vi "InterfaceControladores2.vi"() -> ()   [LabVIEW 2016]
uses:
  <vilib>/Instr/_visa.llb/VISA Configure Serial Port (Instr).vi
panel:
  out "u":dbl
  in  "Tab Control":T1(tab)
  out "Error Signal":dbl(graph)
  out "Control Signal":dbl(graph)
  out "Referece Signal":dbl(graph)
  out "Output Signal":dbl(graph)
  in  "Send":bool
  in  "Fuzzy Input Launcher 2":bool
  in  "Fuzzy Input Launcher":bool
  in  "Send 2":bool
  in  "PORT":refnum<visa-resource-name>
  in  "Controller":u16(ring) items=["On/Off", "On/Off Hysteresis", "Proportional", "Proportional Integral", "Fuzzy", "Open Loop"]
  in  "Reference (V)":dbl(slide) min=0.0 max=20.0 scale=0.0..20.0
  in  "Window Hysteresis %":dbl min=0.0 max=99.0
  in  "Kp":dbl(knob) min=-1.0 max=10.0 scale=-1.0..10.0 scale format="%.1g"
  in  "Ki":dbl(knob) min=0.0 max=10.0 scale=0.0..10.0 scale format="%.1g"
  in  "Stop Button":bool
  out "data sent":string
  out "y":dbl
  # "P/PI Controller"
  # "On/Off with Hysteresis Controller"
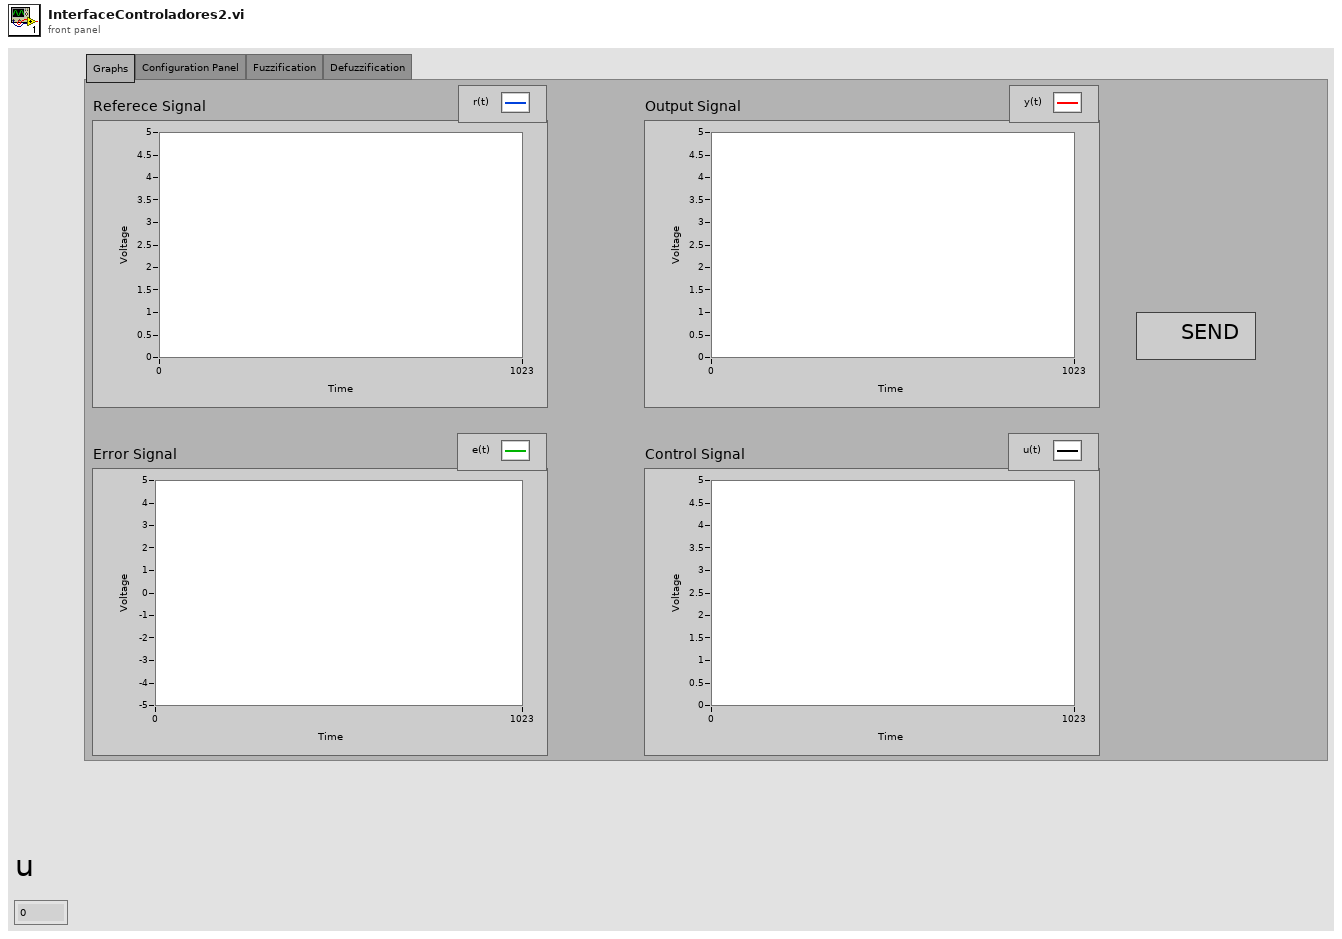
[diagram p1: front panel]
types:
  T1 = enum32{"Graphs", "Configuration Panel", "Fuzzification", "Defuzzification"}
  T2 = enum32{"Invalid", "Standard", "Closed", "Hidden", "Minimized", "Maximized"}
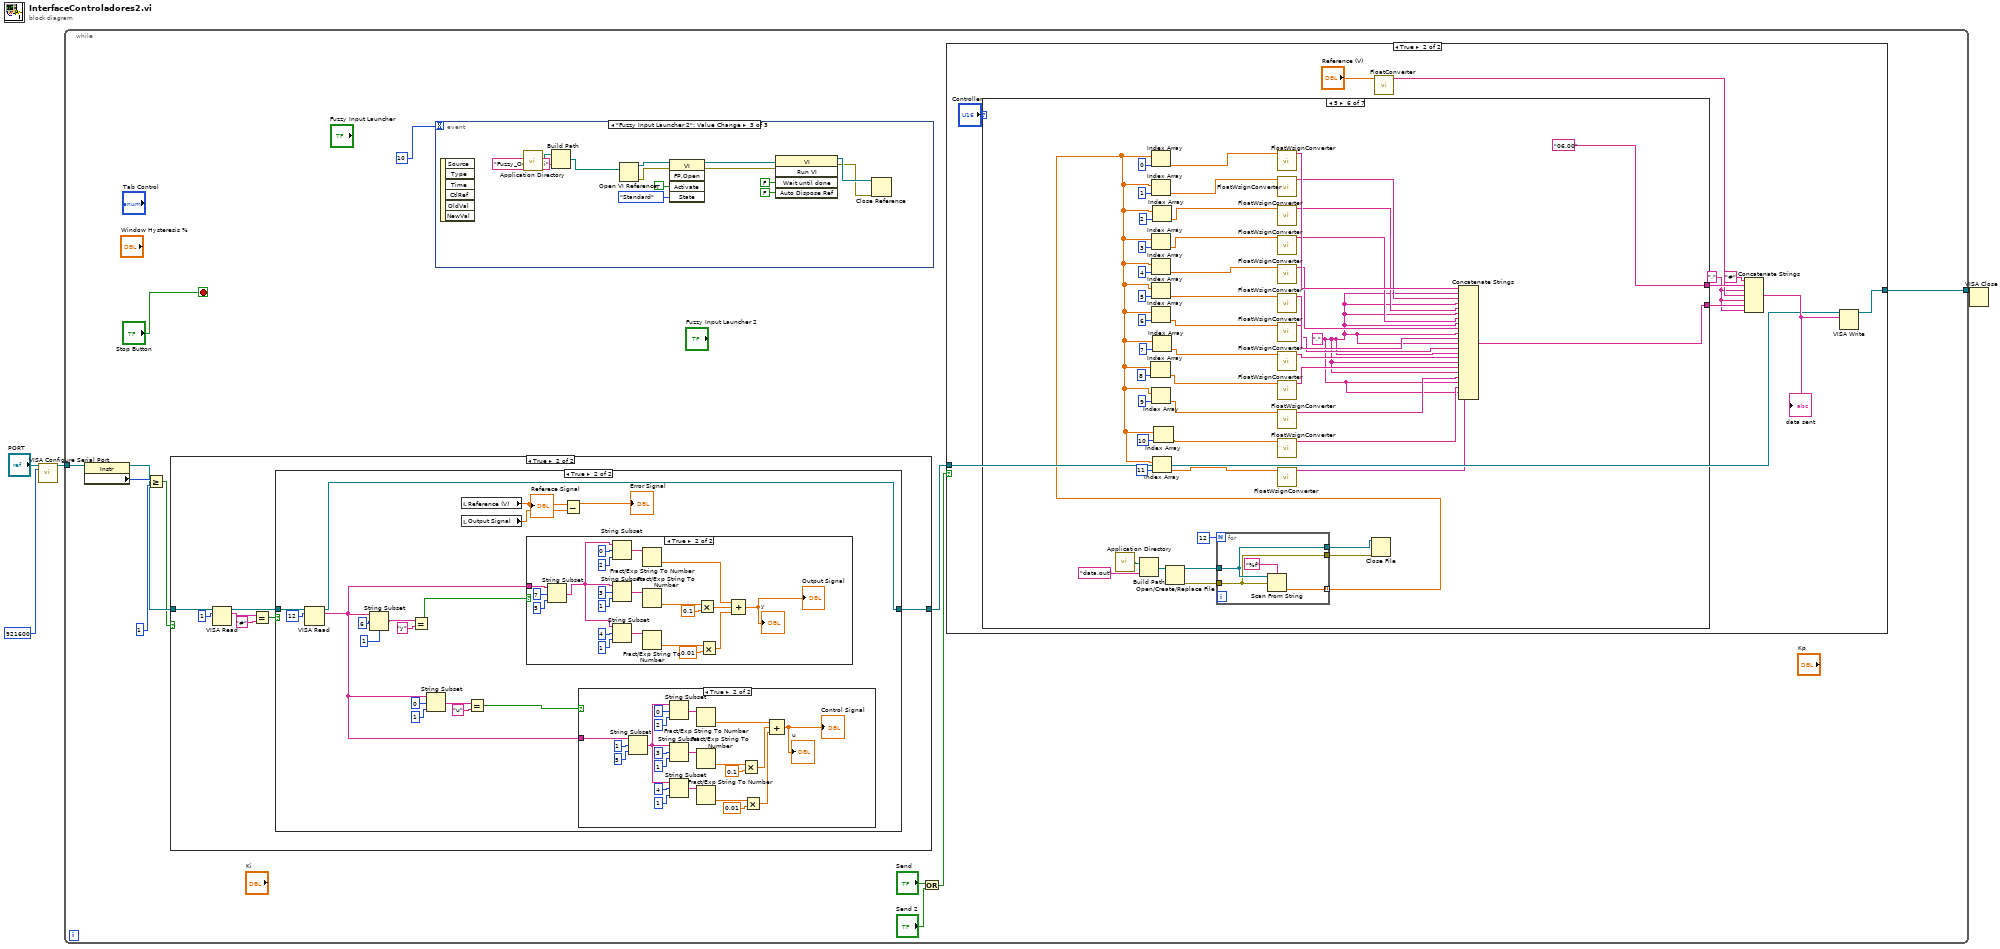
[diagram p0: block diagram]
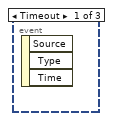
[diagram p2: hidden frame]
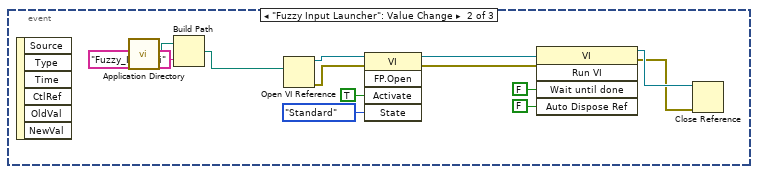
[diagram p3: hidden frame]
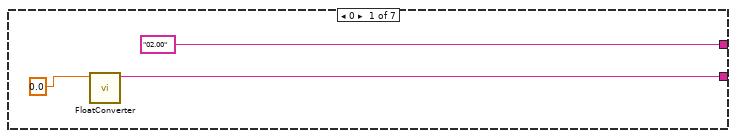
[diagram p9: hidden frame]
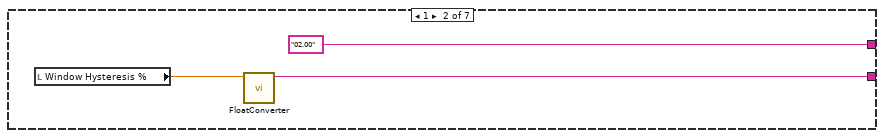
[diagram p10: hidden frame]
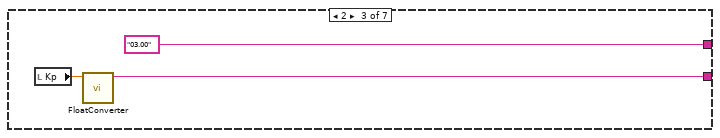
[diagram p11: hidden frame]
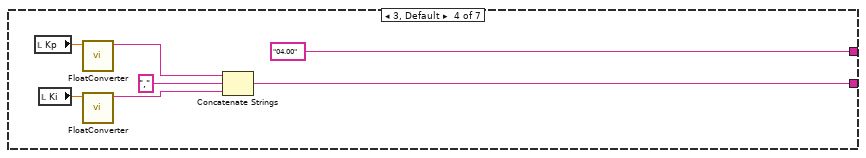
[diagram p12: hidden frame]
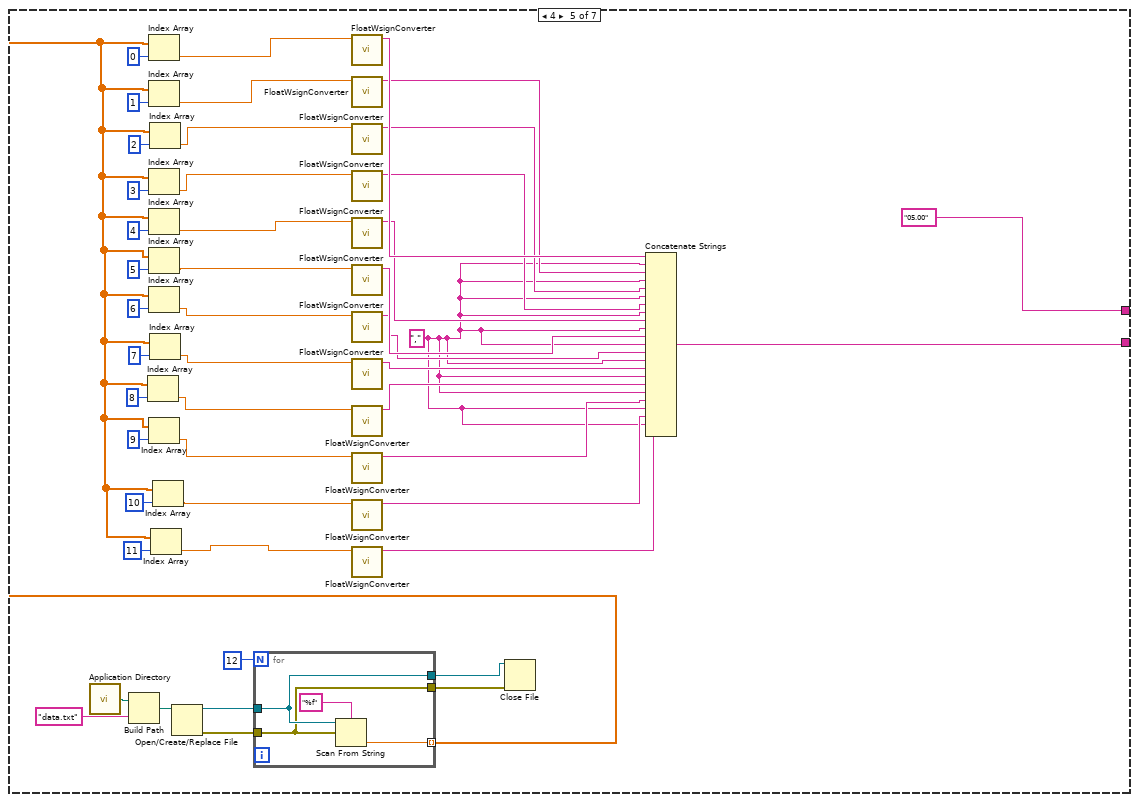
[diagram p13: hidden frame]
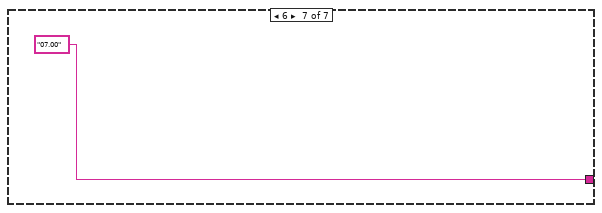
[diagram p14: hidden frame]
diagram:
  n1 = call-poly "VISA Configure Serial Port"("VISA resource name"="PORT", "baud rate (9600)"=u32 921600) -> ("VISA resource name out"=w4:refnum<visa-resource-name>)  [unwired: 12 in, 1 out]
  n2 = while {
    tunnel: w4 -> [w16]
    tunnel: [w13] -> w2
    stop <- "Stop Button" stop-if-true
    n3 = property class="Instr"(reference=w16) -> (reference out=w12:refnum<visa-resource-name>, "Serial Settings:Number of Bytes at Serial Port"=w15:u32)  [unwired: 1 in, 1 out]
    n4 = Greater Or Equal?(x=w15, y=u32 1) -> (x >= y?=w11:bool)
    n5 = case shown="True" w11 {
      tunnel: w12 -> [w43 w50]
      tunnel: [w43 w44] -> w10
      frame False {
      }
      frame True {
        n6 = VISA Read(VISA resource name=w50, byte count=u32 1 ("y")) -> (VISA resource name out=w45:refnum<visa-resource-name>, read buffer=w48:string)  [unwired: 1 in, 2 out]
        n7 = Equal?(x=w48, y="#") -> (x = y?=w46:bool)
        n8 = case shown="True" w46 {
          tunnel: [w51 w67] -> w44
          tunnel: w45 -> [w51 w66]
          frame False {
          }
          frame True {
            n9 = VISA Read(VISA resource name=w66, byte count=u32 12 ("y")) -> (VISA resource name out=w67:refnum<visa-resource-name>, read buffer=w52:string)  [unwired: 1 in, 2 out]
            n10 = String Subset(string=w52, offset (0)=6 ("length (rest)"), length (rest)=1 ("length (rest)")) -> (substring=w55:string)
            n11 = Equal?(x=w55, y="y") -> (x = y?=w54:bool)
            n12 = String Subset(string=w52, offset (0)=0 ("length (rest)"), length (rest)=1 ("length (rest)")) -> (substring=w57:string)
            n13 = local read "Reference (V)"() -> (w64:dbl)
            "Referece Signal" <- w64
            n14 = local read "Output Signal"() -> (w65:dbl)
            n15 = Equal?(x=w57, y="u") -> (x = y?=w53:bool)
            n16 = case shown="True" w54 {
              tunnel: w52 -> [_ w70]
              frame False {
              }
              frame True {
                n17 = String Subset(string=w70, offset (0)=7, length (rest)=5 ("length (rest)")) -> (substring=w69:string)
                n18 = String Subset(string=w69, offset (0)=0, length (rest)=2 ("length (rest)")) -> (substring=w88:string)
                n19 = String Subset(string=w69, offset (0)=3, length (rest)=1 ("length (rest)")) -> (substring=w87:string)
                n20 = String Subset(string=w69, offset (0)=4, length (rest)=1 ("offset (0)")) -> (substring=w79:string)
                n21 = Fract/Exp String To Number(string=w88) -> (number=w76:dbl)  [unwired: 3 in, 1 out]
                n22 = Fract/Exp String To Number(string=w87) -> (number=w84:dbl)  [unwired: 3 in, 1 out]
                n23 = Fract/Exp String To Number(string=w79) -> (number=w80:dbl)  [unwired: 3 in, 1 out]
                n24 = Multiply(x=w84, y=0.1) -> (x*y=w75:dbl)
                n25 = Multiply(x=w80, y=0.01) -> (x*y=w74:dbl)
                n26 = Compound Arithmetic op=ADD(w76, w75, w74) -> (→"Output Signal" →"y":dbl)
              }
            }
            n27 = Subtract(x=w64, y=w65) -> (x-y=→"Error Signal":dbl)
            n28 = case shown="True" w53 {
              tunnel: w52 -> [_ w93]
              frame False {
              }
              frame True {
                n29 = String Subset(string=w93, offset (0)=1, length (rest)=5 ("length (rest)")) -> (substring=w94:string)
                n30 = String Subset(string=w94, offset (0)=0, length (rest)=2 ("offset (0)")) -> (substring=w109:string)
                n31 = String Subset(string=w94, offset (0)=3, length (rest)=1 ("offset (0)")) -> (substring=w107:string)
                n32 = String Subset(string=w94, offset (0)=4, length (rest)=1 ("offset (0)")) -> (substring=w100:string)
                n33 = Fract/Exp String To Number(string=w109) -> (number=w98:dbl)  [unwired: 3 in, 1 out]
                n34 = Fract/Exp String To Number(string=w107) -> (number=w106:dbl)  [unwired: 3 in, 1 out]
                n35 = Fract/Exp String To Number(string=w100) -> (number=w101:dbl)  [unwired: 3 in, 1 out]
                n36 = Multiply(x=w106, y=0.1) -> (x*y=w97:dbl)
                n37 = Multiply(x=w101, y=0.01) -> (x*y=w96:dbl)
                n38 = Compound Arithmetic op=ADD(w98, w97, w96) -> (→"Control Signal" →"u":dbl)
              }
            }
          }
        }
      }
    }
    n39 = event shown="[2] \"Fuzzy Input Launcher 2\": Value Change" {
      selector: _ -> [_ _ _]
      dyn-events: _ -> [_ _ _]
      timeout: 10 -> [_ _ _]
      event Timeout {
        n40 = event-data() -> ()  [unwired: 1 in, 3 out]
      }
      event "Fuzzy Input Launcher": Value Change {
        n41 = event-data() -> ()  [unwired: 1 in, 6 out]
        n42 = call <vilib>:"Application Directory.vi"() -> ("Application Directory"=w29:path)
        n43 = Build Path(base path=w29, name or relative path="Fuzzy_Input.vi") -> (appended path=w27:path)
        n44 = Open VI Reference(vi path=w27) -> (vi reference=w24:refnum<vi>, error out=w23:errorcluster)  [unwired: 5 in]
        n45 = invoke class="VI" method="FP.Open"(reference=w24, error in=w23, "Activate"=TRUE ("Activate?"), "State"=T2."Standard") -> (reference out=w26:refnum<vi>, error out=w25:errorcluster)  [unwired: 1 in, 3 out]
        n46 = invoke class="VI" method="Run VI"(reference=w26, error in=w25, "Wait until done"=FALSE ("Wait Until Done"), "Auto Dispose Ref"=FALSE ("Auto Dispose Reference")) -> (reference out=w18:refnum<vi>, error out=w17:errorcluster)  [unwired: 1 in, 3 out]
        n47 = Close Reference(reference=w18, error in (no error)=w17) -> ()  [unwired: 1 out]
      }
      event "Fuzzy Input Launcher 2": Value Change {
        n48 = event-data() -> ()  [unwired: 1 in, 6 out]
        n49 = call <vilib>:"Application Directory.vi"() -> ("Application Directory"=w42:path)
        n50 = Build Path(base path=w42, name or relative path="Fuzzy_Output.vi") -> (appended path=w40:path)
        n51 = Open VI Reference(vi path=w40) -> (vi reference=w37:refnum<vi>, error out=w36:errorcluster)  [unwired: 5 in]
        n52 = invoke class="VI" method="FP.Open"(reference=w37, error in=w36, "Activate"=TRUE ("Activate?"), "State"=T2."Standard") -> (reference out=w39:refnum<vi>, error out=w38:errorcluster)  [unwired: 1 in, 3 out]
        n53 = invoke class="VI" method="Run VI"(reference=w39, error in=w38, "Wait until done"=FALSE ("Wait Until Done"), "Auto Dispose Ref"=FALSE ("Auto Dispose Reference")) -> (reference out=w31:refnum<vi>, error out=w30:errorcluster)  [unwired: 1 in, 3 out]
        n54 = Close Reference(reference=w31, error in (no error)=w30) -> ()  [unwired: 1 out]
      }
    }
    n55 = Or(x="Send", y="Send 2") -> (x .or. y?=w7:bool)
    n56 = case shown="True" w7 {
      tunnel: [w111 w119] -> w13
      tunnel: w10 -> [w111 w117]
      frame False {
      }
      frame True {
        w112 = ","
        n57 = case shown="5" "Controller" {
          tunnel: [w123 w125 w128 w136 w138 w190 _] -> w113
          tunnel: ["02.00" "02.00" "03.00" "04.00" "05.00" "06.00" "07.00"] -> w115
          frame 0 {
            n58 = call "FloatConverter.vi"("Reference (V)"=0.0) -> ("String"=w123:string)  [unwired: 10 in]
          }
          frame 1 {
            n59 = local read "Window Hysteresis %"() -> (w126:dbl)
            n60 = call "FloatConverter.vi"("Reference (V)"=w126) -> ("String"=w125:string)  [unwired: 10 in]
          }
          frame 2 {
            n61 = local read "Kp"() -> (w129:dbl)
            n62 = call "FloatConverter.vi"("Reference (V)"=w129) -> ("String"=w128:string)  [unwired: 10 in]
          }
          frame 3, Default {
            n63 = local read "Kp"() -> (w134:dbl)
            n64 = local read "Ki"() -> (w132:dbl)
            n65 = call "FloatConverter.vi"("Reference (V)"=w134) -> ("String"=w133:string)  [unwired: 10 in]
            n66 = call "FloatConverter.vi"("Reference (V)"=w132) -> ("String"=w131:string)  [unwired: 10 in]
            n67 = Concatenate Strings(w133, ",", w131) -> (w136:string)
          }
          frame 4 {
            w140 = ","
            n68 = call <vilib>:"Application Directory.vi"() -> ("Application Directory"=w183:path)
            n69 = Build Path(base path=w183, name or relative path="data.txt") -> (appended path=w177:path)
            n70 = Open/Create/Replace File(file path (use dialog)=w177) -> (refnum out=w181:refnum<file>, error out=w180:errorcluster)  [unwired: 5 in, 1 out]
            n71 = for {
              N: 12 -> [_]
              tunnel: w181 -> [w187]
              tunnel: w180 -> [w186]
              tunnel: [w188] -> w164 mode=indexing
              tunnel: [w187] -> w179
              tunnel: [w186] -> w178
              n72 = Scan From String("%f" ("format string"), w187, w186) -> (output 1=w188:dbl)  [unwired: 1 in, 2 out]
            }
            n73 = Index Array(array=w164, index=8) -> (element=w155:dbl)
            n74 = Index Array(array=w164, index=0) -> (element=w163:dbl)
            n75 = Index Array(array=w164, index=1) -> (element=w162:dbl)
            n76 = Index Array(array=w164, index=3) -> (element=w160:dbl)
            n77 = Index Array(array=w164, index=4) -> (element=w159:dbl)
            n78 = Index Array(array=w164, index=5) -> (element=w158:dbl)
            n79 = Index Array(array=w164, index=6) -> (element=w157:dbl)
            n80 = Index Array(array=w164, index=9) -> (element=w154:dbl)
            n81 = Index Array(array=w164, index=2) -> (element=w161:dbl)
            n82 = Index Array(array=w164, index=7) -> (element=w156:dbl)
            n83 = Index Array(array=w164, index=11) -> (element=w152:dbl)
            n84 = Index Array(array=w164, index=10) -> (element=w153:dbl)
            n85 = call "FloatWsignConverter.vi"("Zero Lower Limit"=w163) -> ("String"=w151:string)  [unwired: 10 in]
            n86 = call "FloatWsignConverter.vi"("Zero Lower Limit"=w162) -> ("String"=w150:string)  [unwired: 10 in]
            n87 = call "FloatWsignConverter.vi"("Zero Lower Limit"=w161) -> ("String"=w149:string)  [unwired: 10 in]
            n88 = call "FloatWsignConverter.vi"("Zero Lower Limit"=w160) -> ("String"=w148:string)  [unwired: 10 in]
            n89 = call "FloatWsignConverter.vi"("Zero Lower Limit"=w159) -> ("String"=w147:string)  [unwired: 10 in]
            n90 = call "FloatWsignConverter.vi"("Zero Lower Limit"=w158) -> ("String"=w146:string)  [unwired: 10 in]
            n91 = call "FloatWsignConverter.vi"("Zero Lower Limit"=w157) -> ("String"=w145:string)  [unwired: 10 in]
            n92 = call "FloatWsignConverter.vi"("Zero Lower Limit"=w156) -> ("String"=w144:string)  [unwired: 10 in]
            n93 = call "FloatWsignConverter.vi"("Zero Lower Limit"=w155) -> ("String"=w143:string)  [unwired: 10 in]
            n94 = call "FloatWsignConverter.vi"("Zero Lower Limit"=w154) -> ("String"=w142:string)  [unwired: 10 in]
            n95 = call "FloatWsignConverter.vi"("Zero Lower Limit"=w153) -> ("String"=w141:string)  [unwired: 10 in]
            n96 = call "FloatWsignConverter.vi"("Zero Lower Limit"=w152) -> ("String"=w139:string)  [unwired: 10 in]
            n97 = Close File(refnum=w179, error in=w178) -> ()  [unwired: 2 out]
            n98 = Concatenate Strings(w151, w140, w150, w140, w149, w140, w148, w140, w147, w140, w146, w140, w145, w140, w144, w140, w143, w140, w142, w140, w141, w140, w139) -> (w138:string)
          }
          frame 5 {
            w192 = ","
            n99 = call <vilib>:"Application Directory.vi"() -> ("Application Directory"=w235:path)
            n100 = Build Path(base path=w235, name or relative path="data.out") -> (appended path=w229:path)
            n101 = Open/Create/Replace File(file path (use dialog)=w229) -> (refnum out=w233:refnum<file>, error out=w232:errorcluster)  [unwired: 5 in, 1 out]
            n102 = for {
              N: 12 -> [_]
              tunnel: w233 -> [w239]
              tunnel: w232 -> [w238]
              tunnel: [w240] -> w216 mode=indexing
              tunnel: [w239] -> w231
              tunnel: [w238] -> w230
              n103 = Scan From String("%f" ("format string"), w239, w238) -> (output 1=w240:dbl)  [unwired: 1 in, 2 out]
            }
            n104 = Index Array(array=w216, index=8) -> (element=w207:dbl)
            n105 = Index Array(array=w216, index=0) -> (element=w215:dbl)
            n106 = Index Array(array=w216, index=1) -> (element=w214:dbl)
            n107 = Index Array(array=w216, index=3) -> (element=w212:dbl)
            n108 = Index Array(array=w216, index=4) -> (element=w211:dbl)
            n109 = Index Array(array=w216, index=5) -> (element=w210:dbl)
            n110 = Index Array(array=w216, index=6) -> (element=w209:dbl)
            n111 = Index Array(array=w216, index=9) -> (element=w206:dbl)
            n112 = Index Array(array=w216, index=2) -> (element=w213:dbl)
            n113 = Index Array(array=w216, index=7) -> (element=w208:dbl)
            n114 = Index Array(array=w216, index=11) -> (element=w204:dbl)
            n115 = Index Array(array=w216, index=10) -> (element=w205:dbl)
            n116 = call "FloatWsignConverter.vi"("Zero Lower Limit"=w215) -> ("String"=w203:string)  [unwired: 10 in]
            n117 = call "FloatWsignConverter.vi"("Zero Lower Limit"=w214) -> ("String"=w202:string)  [unwired: 10 in]
            n118 = call "FloatWsignConverter.vi"("Zero Lower Limit"=w213) -> ("String"=w201:string)  [unwired: 10 in]
            n119 = call "FloatWsignConverter.vi"("Zero Lower Limit"=w212) -> ("String"=w200:string)  [unwired: 10 in]
            n120 = call "FloatWsignConverter.vi"("Zero Lower Limit"=w211) -> ("String"=w199:string)  [unwired: 10 in]
            n121 = call "FloatWsignConverter.vi"("Zero Lower Limit"=w210) -> ("String"=w198:string)  [unwired: 10 in]
            n122 = call "FloatWsignConverter.vi"("Zero Lower Limit"=w209) -> ("String"=w197:string)  [unwired: 10 in]
            n123 = call "FloatWsignConverter.vi"("Zero Lower Limit"=w208) -> ("String"=w196:string)  [unwired: 10 in]
            n124 = call "FloatWsignConverter.vi"("Zero Lower Limit"=w207) -> ("String"=w195:string)  [unwired: 10 in]
            n125 = call "FloatWsignConverter.vi"("Zero Lower Limit"=w206) -> ("String"=w194:string)  [unwired: 10 in]
            n126 = call "FloatWsignConverter.vi"("Zero Lower Limit"=w205) -> ("String"=w193:string)  [unwired: 10 in]
            n127 = call "FloatWsignConverter.vi"("Zero Lower Limit"=w204) -> ("String"=w191:string)  [unwired: 10 in]
            n128 = Close File(refnum=w231, error in=w230) -> ()  [unwired: 2 out]
            n129 = Concatenate Strings(w203, w192, w202, w192, w201, w192, w200, w192, w199, w192, w198, w192, w197, w192, w196, w192, w195, w192, w194, w192, w193, w192, w191) -> (w190:string)
          }
          frame 6 {
          }
        }
        n130 = call "FloatConverter.vi"("Reference (V)"="Reference (V)") -> ("String"=w114:string)  [unwired: 10 in]
        n131 = Concatenate Strings("#" ("string"), w115, w112, w114, w112, w113, w112) -> (w120:string)
        "data sent" <- w120
        n132 = VISA Write(VISA resource name=w117, write buffer=w120) -> (VISA resource name out=w119:refnum<visa-resource-name>)  [unwired: 1 in, 2 out]
      }
    }
  }
  n133 = VISA Close(VISA resource name=w2) -> ()  [unwired: 1 in, 1 out]
